vi "TTA_MATLAB_TX_OutputPowerTest_DetailedResults.vi"(8 "error in":errorcluster, 9 "Tx Output \nPower Results":T1(array[cluster]), 10 "TestGroup":string, 11 "SubTest":string) -> (0 "error out":errorcluster, 3 "SubTestSuccess":dbl[](array[numeric]))   [LabVIEW 2016]
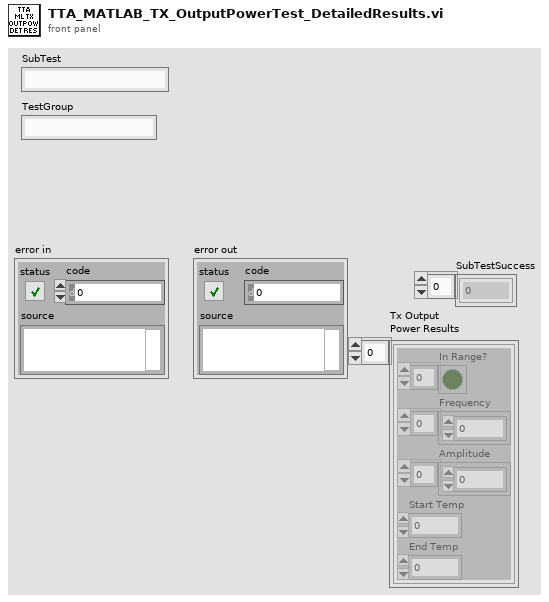
[diagram p1: front panel]
types:
  T1 = cluster{"In Range?":bool[], "Frequency":dbl[], "Amplitude":dbl[], "Start Temp":dbl, "End Temp":dbl}[]
  T2 = cluster{"In Range?":bool[], "Frequency":dbl[], "Amplitude":dbl[], "Start Temp":dbl, "End Temp":dbl}
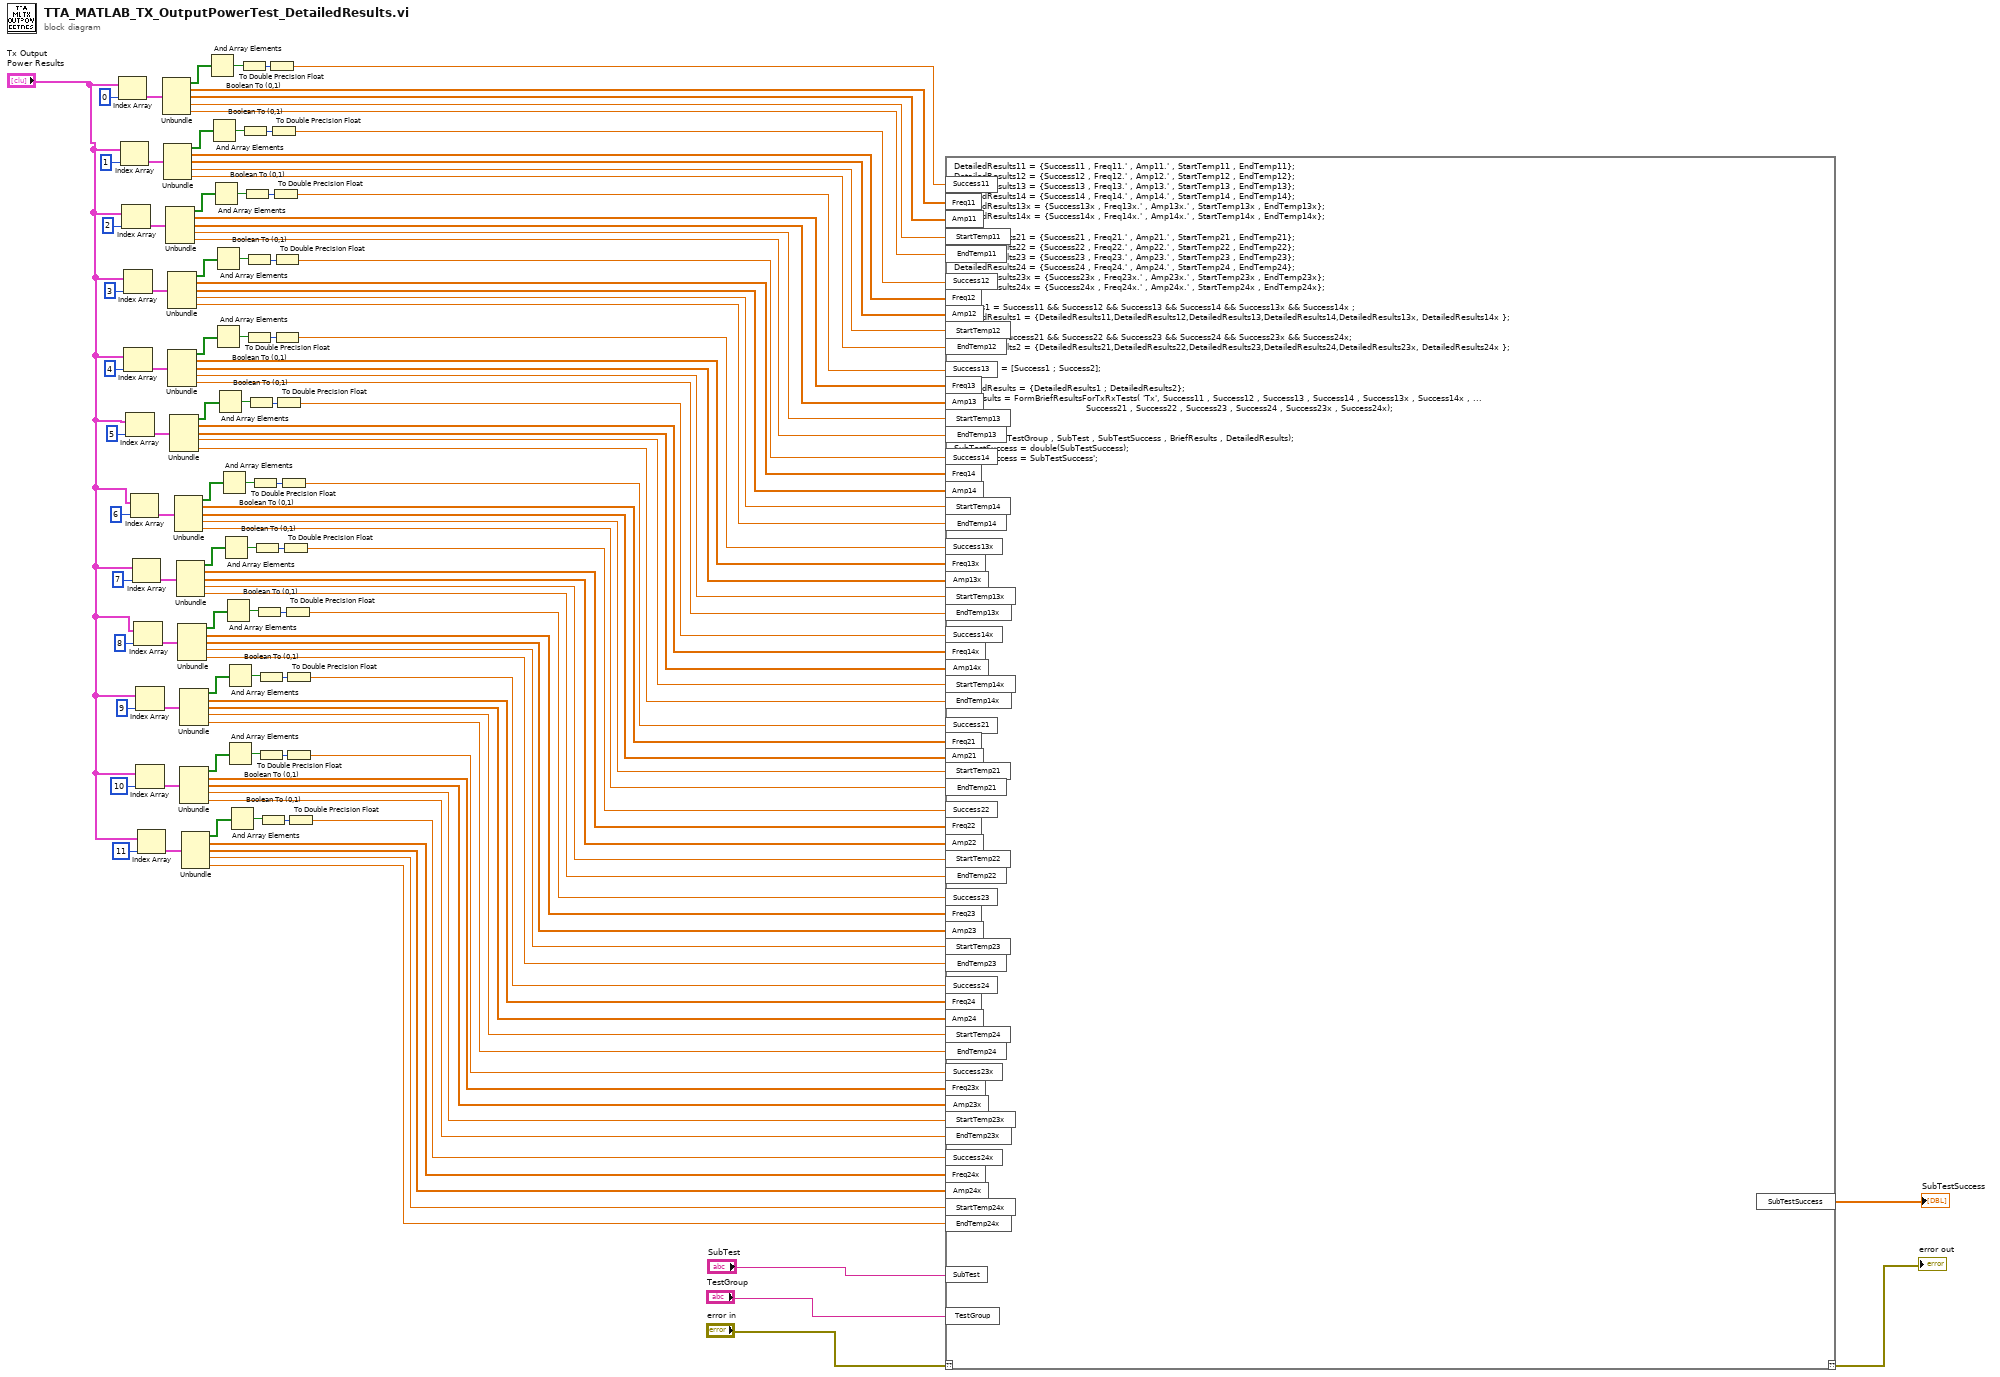
[diagram p0: block diagram]
diagram:
  (unwired) 5 ("index")
  (unwired) 3 ("index")
  (unwired) 2 ("index")
  (unwired) 1 ("index")
  (unwired) 0 ("index")
  (unwired) 5 ("index")
  (unwired) 4 ("index")
  (unwired) 3 ("index")
  (unwired) 2 ("index")
  (unwired) 1 ("index")
  (unwired) 0 ("index")
  (unwired) 5 ("index")
  (unwired) 4 ("index")
  (unwired) 3 ("index")
  (unwired) 2 ("index")
  (unwired) 1 ("index")
  (unwired) 0 ("index")
  (unwired) 5 ("index")
  (unwired) 4 ("index")
  (unwired) 3 ("index")
  (unwired) 2 ("index")
  (unwired) 1 ("index")
  (unwired) 0 ("index")
  (unwired) 4 ("index")
  n1 = Index Array(array="Tx Output \nPower Results", index=0) -> (element=w6:T2)
  n2 = Index Array(array="Tx Output \nPower Results", index=1) -> (element=w16:T2)
  n3 = Index Array(array="Tx Output \nPower Results", index=2) -> (element=w15:T2)
  n4 = Index Array(array="Tx Output \nPower Results", index=3) -> (element=w14:T2)
  n5 = Index Array(array="Tx Output \nPower Results", index=4) -> (element=w73:T2)
  n6 = Index Array(array="Tx Output \nPower Results", index=5) -> (element=w12:T2)
  n7 = Index Array(array="Tx Output \nPower Results", index=6) -> (element=w79:T2)
  n8 = Index Array(array="Tx Output \nPower Results", index=7) -> (element=w78:T2)
  n9 = Index Array(array="Tx Output \nPower Results", index=8) -> (element=w43:T2)
  n10 = Index Array(array="Tx Output \nPower Results", index=9) -> (element=w37:T2)
  n11 = Index Array(array="Tx Output \nPower Results", index=10) -> (element=w35:T2)
  n12 = Index Array(array="Tx Output \nPower Results", index=11) -> (element=w33:T2)
  n13 = Unbundle(w6) -> ("In Range?"=w5:bool[], "Frequency"=w4:dbl[], "Amplitude"=w3:dbl[], "Start Temp"=w2:dbl, "End Temp"=w1:dbl)
  n14 = Unbundle(w16) -> ("In Range?"=w11:bool[], "Frequency"=w64:dbl[], "Amplitude"=w63:dbl[], "Start Temp"=w62:dbl, "End Temp"=w61:dbl)
  n15 = Unbundle(w15) -> ("In Range?"=w10:bool[], "Frequency"=w60:dbl[], "Amplitude"=w59:dbl[], "Start Temp"=w58:dbl, "End Temp"=w57:dbl)
  n16 = Unbundle(w14) -> ("In Range?"=w9:bool[], "Frequency"=w68:dbl[], "Amplitude"=w67:dbl[], "Start Temp"=w66:dbl, "End Temp"=w65:dbl)
  n17 = Unbundle(w73) -> ("In Range?"=w8:bool[], "Frequency"=w72:dbl[], "Amplitude"=w71:dbl[], "Start Temp"=w70:dbl, "End Temp"=w69:dbl)
  n18 = Unbundle(w12) -> ("In Range?"=w7:bool[], "Frequency"=w77:dbl[], "Amplitude"=w76:dbl[], "Start Temp"=w75:dbl, "End Temp"=w74:dbl)
  n19 = Unbundle(w79) -> ("In Range?"=w56:bool[], "Frequency"=w54:dbl[], "Amplitude"=w53:dbl[], "Start Temp"=w52:dbl, "End Temp"=w51:dbl)
  n20 = Unbundle(w78) -> ("In Range?"=w50:bool[], "Frequency"=w48:dbl[], "Amplitude"=w47:dbl[], "Start Temp"=w46:dbl, "End Temp"=w45:dbl)
  n21 = Unbundle(w43) -> ("In Range?"=w44:bool[], "Frequency"=w41:dbl[], "Amplitude"=w40:dbl[], "Start Temp"=w39:dbl, "End Temp"=w38:dbl)
  n22 = Unbundle(w37) -> ("In Range?"=w36:bool[], "Frequency"=w30:dbl[], "Amplitude"=w29:dbl[], "Start Temp"=w28:dbl, "End Temp"=w27:dbl)
  n23 = Unbundle(w35) -> ("In Range?"=w34:bool[], "Frequency"=w25:dbl[], "Amplitude"=w24:dbl[], "Start Temp"=w23:dbl, "End Temp"=w22:dbl)
  n24 = Unbundle(w33) -> ("In Range?"=w32:bool[], "Frequency"=w20:dbl[], "Amplitude"=w19:dbl[], "Start Temp"=w18:dbl, "End Temp"=w17:dbl)
  n25 = And Array Elements(Boolean array=w5) -> (logical AND=w120:bool)
  n26 = And Array Elements(Boolean array=w11) -> (logical AND=w116:bool)
  n27 = And Array Elements(Boolean array=w10) -> (logical AND=w109:bool)
  n28 = And Array Elements(Boolean array=w9) -> (logical AND=w112:bool)
  n29 = And Array Elements(Boolean array=w8) -> (logical AND=w107:bool)
  n30 = And Array Elements(Boolean array=w7) -> (logical AND=w104:bool)
  n31 = And Array Elements(Boolean array=w56) -> (logical AND=w81:bool)
  n32 = And Array Elements(Boolean array=w50) -> (logical AND=w84:bool)
  n33 = And Array Elements(Boolean array=w44) -> (logical AND=w90:bool)
  n34 = And Array Elements(Boolean array=w36) -> (logical AND=w87:bool)
  n35 = And Array Elements(Boolean array=w34) -> (logical AND=w93:bool)
  n36 = And Array Elements(Boolean array=w32) -> (logical AND=w96:bool)
  n37 = Boolean To (0,1)(Boolean=w120) -> (0, 1=w119:i16)
  n38 = Boolean To (0,1)(Boolean=w116) -> (0, 1=w117:i16)
  n39 = Boolean To (0,1)(Boolean=w109) -> (0, 1=w110:i16)
  n40 = Boolean To (0,1)(Boolean=w112) -> (0, 1=w111:i16)
  n41 = Boolean To (0,1)(Boolean=w107) -> (0, 1=w106:i16)
  n42 = Boolean To (0,1)(Boolean=w104) -> (0, 1=w105:i16)
  n43 = Boolean To (0,1)(Boolean=w81) -> (0, 1=w82:i16)
  n44 = Boolean To (0,1)(Boolean=w84) -> (0, 1=w83:i16)
  n45 = Boolean To (0,1)(Boolean=w90) -> (0, 1=w89:i16)
  n46 = Boolean To (0,1)(Boolean=w87) -> (0, 1=w88:i16)
  n47 = Boolean To (0,1)(Boolean=w93) -> (0, 1=w94:i16)
  n48 = Boolean To (0,1)(Boolean=w96) -> (0, 1=w95:i16)
  n49 = To Double Precision Float(number=w119) -> (double precision float=w118:dbl)
  n50 = To Double Precision Float(number=w117) -> (double precision float=w114:dbl)
  n51 = To Double Precision Float(number=w110) -> (double precision float=w102:dbl)
  n52 = To Double Precision Float(number=w111) -> (double precision float=w101:dbl)
  n53 = To Double Precision Float(number=w106) -> (double precision float=w100:dbl)
  n54 = To Double Precision Float(number=w105) -> (double precision float=w99:dbl)
  n55 = To Double Precision Float(number=w82) -> (double precision float=w55:dbl)
  n56 = To Double Precision Float(number=w83) -> (double precision float=w49:dbl)
  n57 = To Double Precision Float(number=w89) -> (double precision float=w42:dbl)
  n58 = To Double Precision Float(number=w88) -> (double precision float=w31:dbl)
  n59 = To Double Precision Float(number=w94) -> (double precision float=w26:dbl)
  n60 = To Double Precision Float(number=w95) -> (double precision float=w21:dbl)
  n61 = script code="DetailedResults11 = {Success11 , Freq11.' , Amp11.' , StartTemp11 , EndTemp11};\nDetailedResults12 = {Success12 , Freq12.' , Amp12.' , StartTemp12 , EndTemp12};\nDetailedResults13 = {Success13 , Freq13.' , Amp13.' , StartTemp13 , EndTemp13};\nDetailedResults14 = {Success14 , Freq14.' , Amp14.' , StartTemp14 , EndTemp14};\nDetailedResults13x = {Success13x , Freq13x.' , Amp13x.' , StartTemp13x , EndTemp13x};\nDetailedResults14x = {Success14x , Freq14x.' , Amp14x.' , StartTemp14x , EndTemp14x};\n\nDetailedResults21 = {Success21 , Freq21.' , Amp21.' , StartTemp21 , EndTemp21};\nDetailedResults22 = {Success22 , Freq22.' , Amp22.' , StartTemp22 , EndTemp22};\nDetailedResults23 = {Success23 , Freq23.' , Amp23.' , StartTemp23 , EndTemp23};\nDetailedResults24 = {Success24 , Freq24.' , Amp24.' , StartTemp24 , EndTemp24};\nDetailedResults23x = {Success23x , Freq23x.' , Amp23x.' , StartTemp23x , EndTemp23x};\nDetailedResults24x = {Success24x , Freq24x.' , Amp24x.' , StartTemp24x , EndTemp24x};\n\nSuccess1 = Success11 && Success12 && Success13 && Success14 && Success13x && Success14x ;\nDetailedResults1 = {DetailedResults11,DetailedResults12,DetailedResults13,DetailedResults14,DetailedResults13x, DetailedResults14x };\n\nSuccess2 = Success21 && Success22 && Success23 && Success24 && Success23x && Success24x;\nDetailedResults2 = {DetailedResults21,DetailedResults22,DetailedResults23,DetailedResults24,DetailedResults23x, DetailedResults24x };\n\nSuccessList = [Success1 ; Success2];\n\nDetailedResults = {DetailedResults1 ; DetailedResults2};\nBriefResults = FormBriefResultsForTxRxTests( 'Tx', Success11 , Success12 , Success13 , Success14 , Success13x , Success14x , ...\n                                            Success21 , Success22 , Success23 , Success24 , Success23x , Success24x);\n\n\nUpdateState(TestGroup , SubTest , SubTestSuccess , BriefResults , DetailedResults);\nSubTestSuccess = double(SubTestSuccess);\nSubTestSuccess = SubTestSuccess';"("??"="error in", "SubTest"="SubTest", "TestGroup"="TestGroup", "Success11"=w118, "Freq11"=w4, "Amp11"=w3, "StartTemp11"=w2, "EndTemp11"=w1, "Success12"=w114, "Freq12"=w64, "Amp12"=w63, "StartTemp12"=w62, "EndTemp12"=w61, "Success13"=w102, "Freq13"=w60, "Amp13"=w59, "StartTemp13"=w58, "EndTemp13"=w57, "Success14"=w101, "Freq14"=w68, "Amp14"=w67, "StartTemp14"=w66, "EndTemp14"=w65, "Success13x"=w100, "Freq13x"=w72, "Amp13x"=w71, "StartTemp13x"=w70, "EndTemp13x"=w69, "Success14x"=w99, "Freq14x"=w77, "Amp14x"=w76, "StartTemp14x"=w75, "EndTemp14x"=w74, "Success21"=w55, "Freq21"=w54, "Amp21"=w53, "StartTemp21"=w52, "EndTemp21"=w51, "Success22"=w49, "Freq22"=w48, "Amp22"=w47, "StartTemp22"=w46, "EndTemp22"=w45, "Success23"=w42, "Freq23"=w41, "Amp23"=w40, "StartTemp23"=w39, "EndTemp23"=w38, "Success24"=w31, "Freq24"=w30, "Amp24"=w29, "StartTemp24"=w28, "EndTemp24"=w27, "Success23x"=w26, "Freq23x"=w25, "Amp23x"=w24, "StartTemp23x"=w23, "EndTemp23x"=w22, "Success24x"=w21, "Freq24x"=w20, "Amp24x"=w19, "StartTemp24x"=w18, "EndTemp24x"=w17) -> ("??"=→"error out":errorcluster, "SubTestSuccess"=→"SubTestSuccess":dbl[])
